vi "存储数据.vi"(8 "error in (no error)":errorcluster caption="错误输入（无错误）", 11 "LS-H600-TCP Client 输入":refnum<class "LS-H600-TCP Client.lvclass">) -> (0 "error out":errorcluster caption="错误输出", 3 "LS-H600-TCP Client 输出":refnum<class "LS-H600-TCP Client.lvclass">)   [LabVIEW 2022 SP3, in "LS-H600-TCP Client.lvlib" / "LS-H600-TCP Client.lvclass"]
uses:
  LS-H600-TCP Client.lvclass
  LS-H600-TCP Client.lvclass/LS-H600-TCP Client.ctl
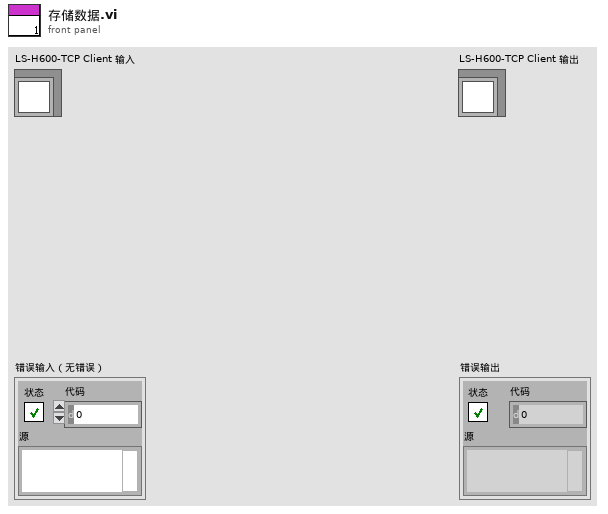
[diagram p1: front panel]
types:
  T1 = cluster{"数据输出":string, "data":cluster{"时间":timestamp, "仪器水深":dbl, "水温":dbl, "流速":dbl, "过水面积":dbl, "瞬时流量":dbl, "累积流量":dbl, "剖面流速":dbl[]}, "连接错误":errorcluster}
  T2 = cluster{"时间":timestamp, "仪器水深":dbl, "水温":dbl, "流速":dbl, "过水面积":dbl, "瞬时流量":dbl, "累积流量":dbl, "剖面流速":dbl[]}
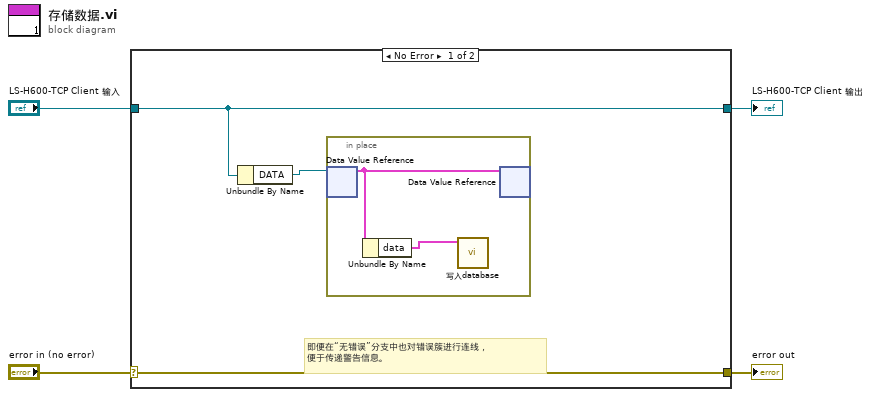
[diagram p0: block diagram]
diagram:
  n1 = case shown="No Error" "error in (no error)" {
    selector: "error in (no error)" -> [w7 w11]
    tunnel: [w7 w11] -> w3
    tunnel: [w6 w10] -> w1
    tunnel: "LS-H600-TCP Client 输入" -> [w6 w10]
    frame No Error {
      # "即便在“无错误”分支中也对错误簇进行连线，\n便于传递警告信息。"
      n2 = Unbundle By Name(w6) -> ("DATA"=w5:refnum<data-value>)
      n3 = in-place {
        n4 = in-place-dvr #1(w5) -> (w9:T1)  [unwired: 1 out]
        n5 = Unbundle By Name(w9) -> ("data"=w8:T2)
        n6 = call "写入database.vi"("data"=w8) -> ()  [unwired: 10 in, 1 out]
        n7 = in-place-dvr #1(w9) -> ()  [unwired: 2 out]
      }
    }
    frame Error {
    }
  }
  "error out" <- w3
  "LS-H600-TCP Client 输出" <- w1
